vi "ArmFrameLimit.vi"(9 "Extend Setpoint":dbl, 10 "Lift Setpoint":dbl) -> (2 "Extend Position":dbl, 3 "Lift Setpoint":dbl)   [LabVIEW 2020]
uses:
  <vilib>/Rock Robotics/WPI/ThirdParty/JAS_Junk/TrajLib/Trajectory_Library.lvlib
  <vilib>/Rock Robotics/WPI/ThirdParty/JAS_Junk/TrajLib/TypeDef/X_Y_PAIR.ctl
panel:
  in  "Extend Position":dbl
  in  "Lift Position":dbl
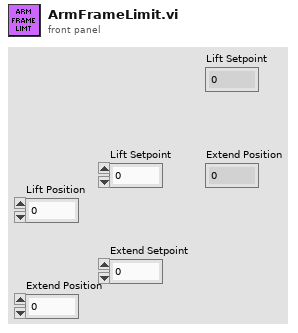
[diagram p1: front panel]
types:
  T1 = typedef "Trajectory_Library.lvlib/X_Y_PAIR.ctl" = cluster{"X":dbl, "Y":dbl}
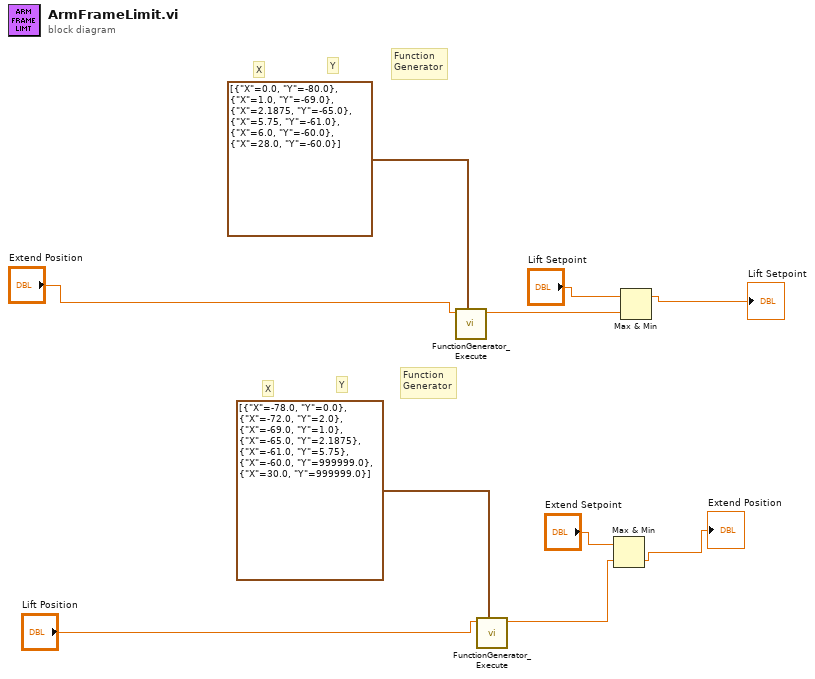
[diagram p0: block diagram]
diagram:
  # "Function\nGenerator"
  # "Y"
  # "X"
  # "Function\nGenerator"
  # "Y"
  # "X"
  n1 = call <vilib>:"FunctionGenerator_Execute.vi"("X Y Pairs"=T1[] [{"X"=0.0, "Y"=-80.0}, {"X"=1.0, "Y"=-69.0}, {"X"=2.1875, "Y"=-65.0}, {"X"=5.75, "Y"=-61.0}, {"X"=6.0, "Y"=-60.0}, {"X"=28.0, "Y"=-60.0}], "Input Value"="Extend Position") -> ("Output Value"=w6:dbl)  [unwired: 9 in]
  n2 = call <vilib>:"FunctionGenerator_Execute.vi"("X Y Pairs"=T1[] [{"X"=-78.0, "Y"=0.0}, {"X"=-72.0, "Y"=2.0}, {"X"=-69.0, "Y"=1.0}, {"X"=-65.0, "Y"=2.1875}, {"X"=-61.0, "Y"=5.75}, {"X"=-60.0, "Y"=999999.0}, {"X"=30.0, "Y"=999999.0}], "Input Value"="Lift Position") -> ("Output Value"=w2:dbl)  [unwired: 9 in]
  n3 = Max & Min(x="Extend Setpoint", y=w2) -> (min(x,y)=→"Extend Position":dbl)  [unwired: 1 out]
  n4 = Max & Min(x="Lift Setpoint", y=w6) -> (max(x,y)=→"Lift Setpoint":dbl)  [unwired: 1 out]
